vi "SetOrigin.vi"(7 "Available Points in":refnum<vi>, 8 "Error In":errorcluster, 11 "CoordinatteEntry In":T1 {"CaliperSetting"."CaliperEntry"."CaliperType" items=["Distance", "Mid Point", "Perpendicular Projection", "Lines Intersection", "Angle from Horizontal", "Angle from Vertical", "Angle Defined by 3 Points", "Angle Defined by 4 Points", "Bissecting Line", "Mid Line", "Center of Mass", "Area", "Line Fit", "Circle Fit", "Ellipse Fit"]; "OriginPointInfo"."Mode" items=["Horizontal Motion", "Vertical Motion", "Horizontal and Vertical Motion", "Horizontal. Vertical and Angular Motion"]; "AnalysisSetting"."ROI"."Contours"."Type" items=["No Selection", "Point", "Line", "Rectangle", "Oval", "Polygon", "Freehand Region", "Annulus", "Unused2", "Unused3", "Broken Line", "Freehand Line", "Rotated Rectangle"]}) -> (0 "Error Out":errorcluster, 1 "OriginSet?":bool, 3 "CoordinatteEntry Out":T1 {"CaliperSetting"."CaliperEntry"."CaliperType" items=["Distance", "Mid Point", "Perpendicular Projection", "Lines Intersection", "Angle from Horizontal", "Angle from Vertical", "Angle Defined by 3 Points", "Angle Defined by 4 Points", "Bissecting Line", "Mid Line", "Center of Mass", "Area", "Line Fit", "Circle Fit", "Ellipse Fit"]; "OriginPointInfo"."Mode" items=["Horizontal Motion", "Vertical Motion", "Horizontal and Vertical Motion", "Horizontal. Vertical and Angular Motion"]; "AnalysisSetting"."ROI"."Contours"."Type" items=["No Selection", "Point", "Line", "Rectangle", "Oval", "Polygon", "Freehand Region", "Annulus", "Unused2", "Unused3", "Broken Line", "Freehand Line", "Rotated Rectangle"]})   [LabVIEW 2015]
uses:
  Control/CoordinatteEntry.ctl
  Process/Controls/Process_Setting.ctl
  Process/Controls/Process_Type.ctl
  Control/CoordinateAnalysisSetting.ctl
  Control/CoordinateCaliperSetting.ctl
  Caliper/Controls/CaliperDataEntry.ctl
  Caliper/Controls/CaliperType.ctl
  Caliper/Controls/SelectionListEntry.ctl
  Caliper/Controls/SelectionListEntryPointType.ctl
  Caliper/Controls/CaliperResult.ctl
  <vilib>/Utility/miscctls.llb/LVRowAndColumnTypeDef.ctl
panel:
  in  "Mode":u16(ring) items=["Horizontal Motion", "Vertical Motion", "Horizontal and Vertical Motion", "Horizontal. Vertical and Angular Motion"]
  in  "Cancel":bool
  in  "Done":bool
  in  "Available Points":i32(listbox)=5
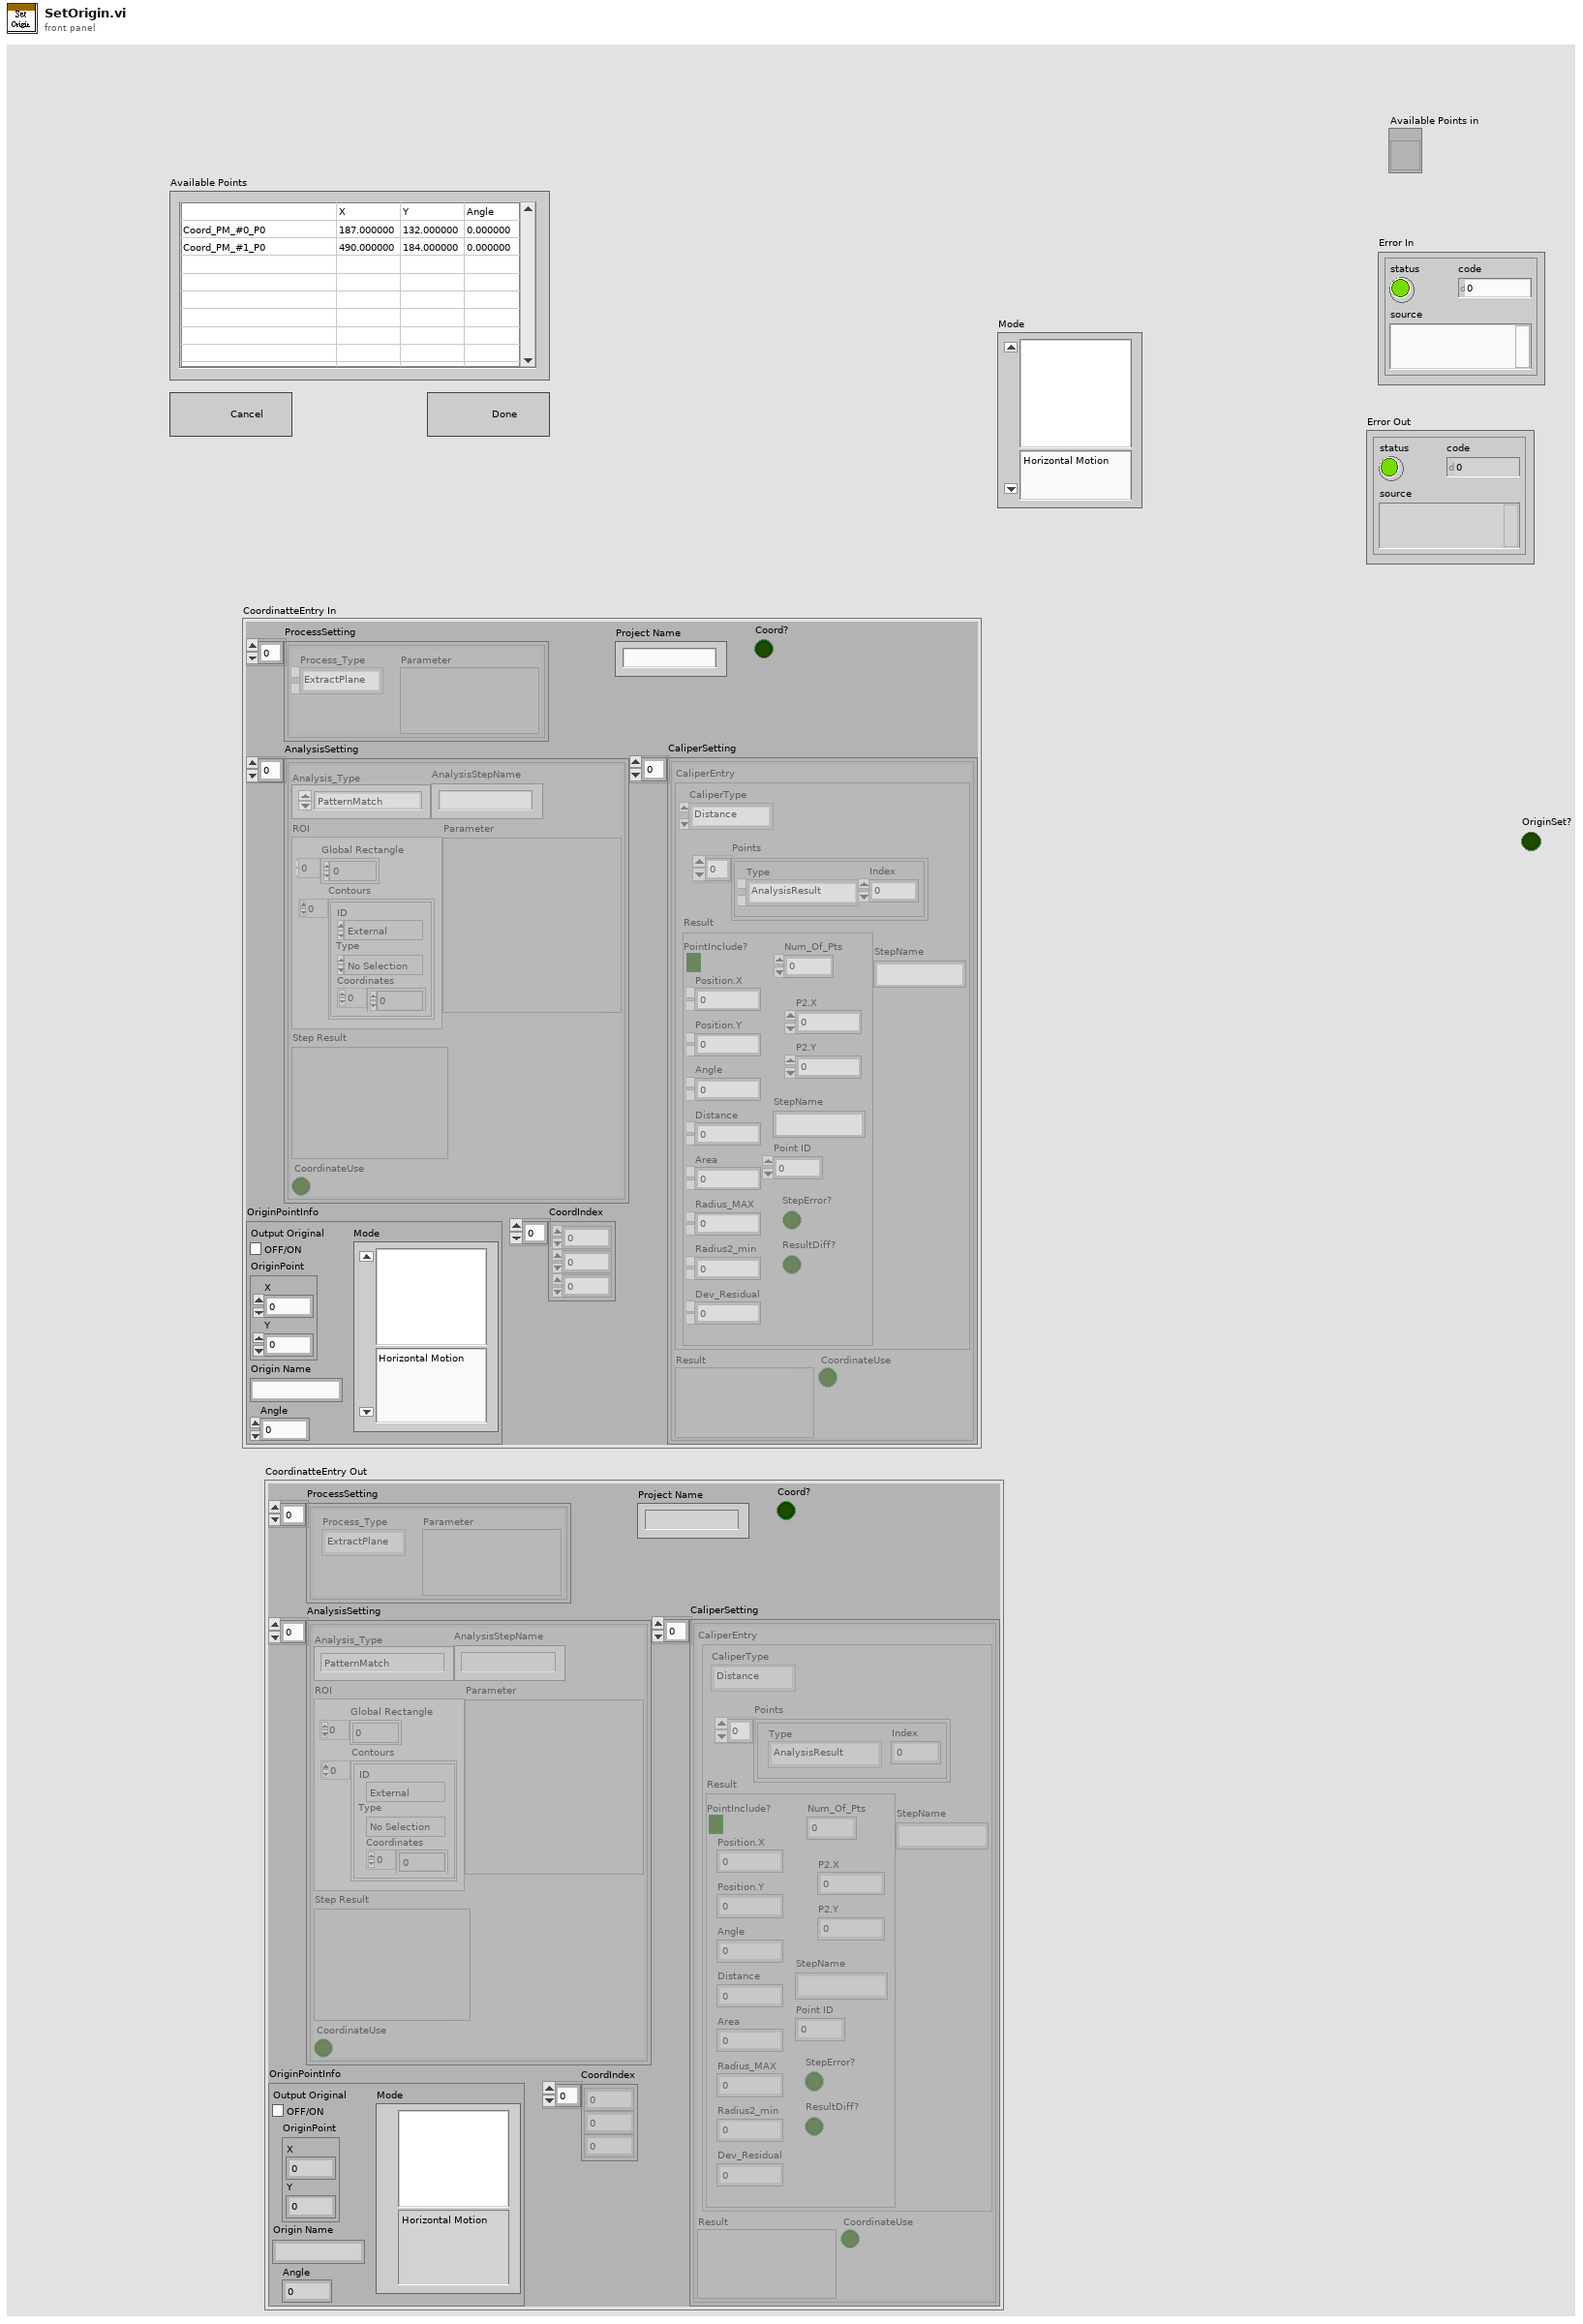
[diagram p1: front panel]
types:
  T1 = typedef "CoordinatteEntry.ctl" = cluster{"ProcessSetting":T2[], "Project Name":string, "AnalysisSetting":T4[], "Coord?":bool, "OriginPointInfo":cluster{"Output Original":bool, "Origin Name":string, "Angle":dbl, "Mode":u16, "OriginPoint":cluster{"X":dbl, "Y":dbl}}, "CaliperSetting":T6[], "CoordIndex":i32[]}
  T2 = typedef "Process_Setting.ctl" = cluster{"Process_Type":T3, "Parameter":variant}
  T3 = typedef "Process_Type.ctl" = enum16{"None", "ExtractPlane", "BinaryMono", "Operators", "GrayMorphology", "Filters", "Lookup Table", "Particle Filter", "Mask"}
  T4 = typedef "CoordinateAnalysisSetting.ctl" = cluster{"Analysis_Type":enum16{"PatternMatch", "Straight Edge"}, "ROI ":T5, "Parameter":variant, "Step Result":variant, "AnalysisStepName":string, "CoordinateUse":bool}
  T5 = typedef "ROI Descriptor" = cluster{"Global Rectangle":i32[], "Contours":cluster{"ID":enum32{"External", "Internal"}, "Type":u32, "Coordinates":i32[]}[]}
  T6 = typedef "CoordinateCaliperSetting.ctl" = cluster{"Result":variant, "CoordinateUse":bool, "CaliperEntry":T7}
  T7 = typedef "CaliperDataEntry.ctl" = cluster{"CaliperType":T8, "Points":T9[], "Result":T11, "StepName":string}
  T8 = typedef "CaliperType.ctl" = u32
  T9 = typedef "SelectionListEntry.ctl" = cluster{"Type":T10, "Index":i32}
  T10 = typedef "SelectionListEntryPointType.ctl" = enum16{"AnalysisResult", "CaliperResult"}
  T11 = typedef "CaliperResult.ctl" = cluster{"PointInclude?":bool, "Num_Of_Pts":u8, "Position.X":dbl, "Position.Y":dbl, "Angle":dbl, "Distance":dbl, "Area":dbl, "Radius_MAX":dbl, "Radius2_min":dbl, "Dev_Residual":dbl, "P2.X":dbl, "P2.Y":dbl, "StepName":string, "Point ID":u8, "StepError?":bool, "ResultDiff?":bool}
  T12 = typedef "LVRowAndColumnTypeDef.ctl" = cluster{"Row":i32, "Column":i32}
  T13 = cluster{"Output Original":bool, "Origin Name":string, "Angle":dbl, "Mode":u16, "OriginPoint":cluster{"X":dbl, "Y":dbl}}
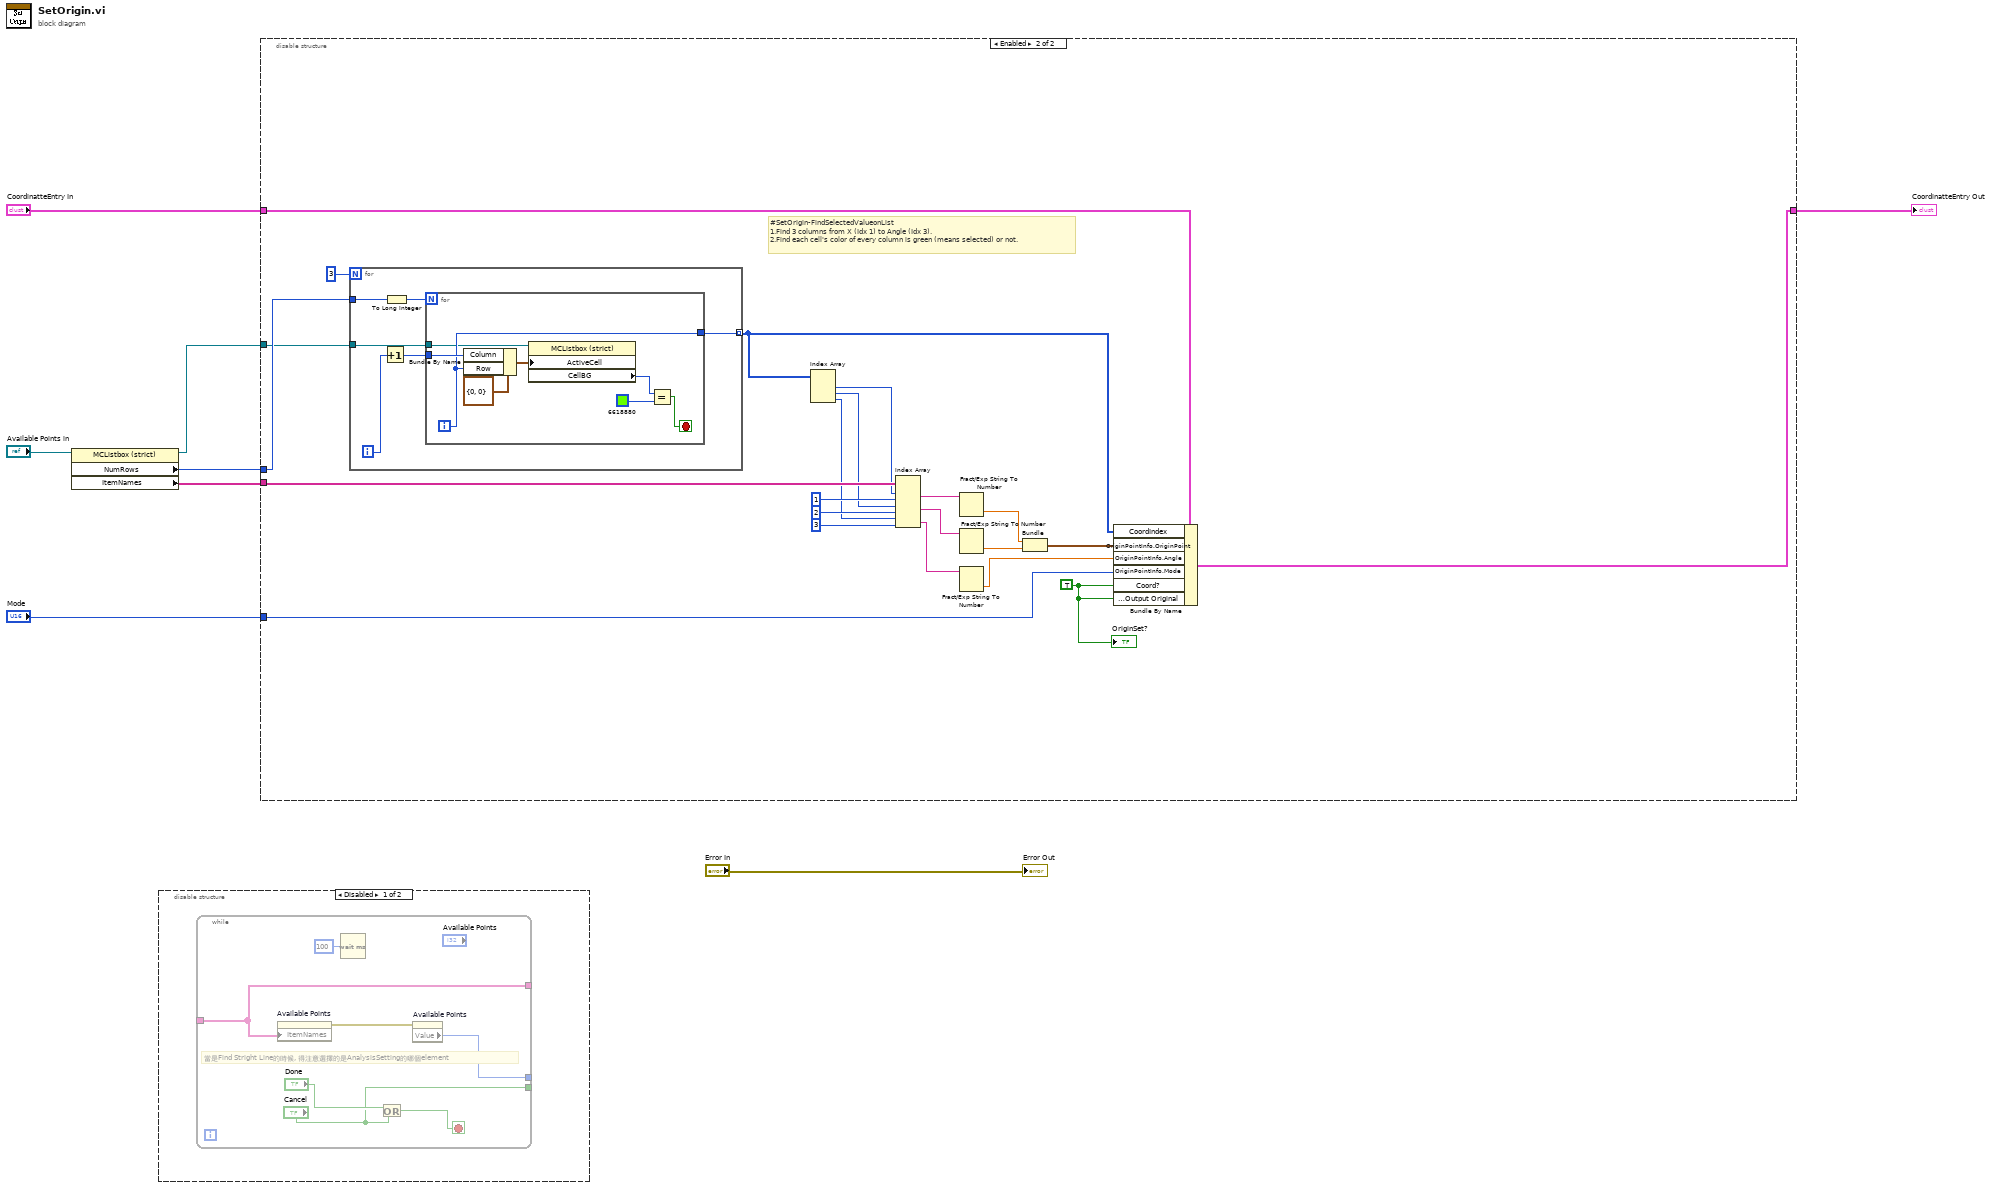
[diagram p0: block diagram]
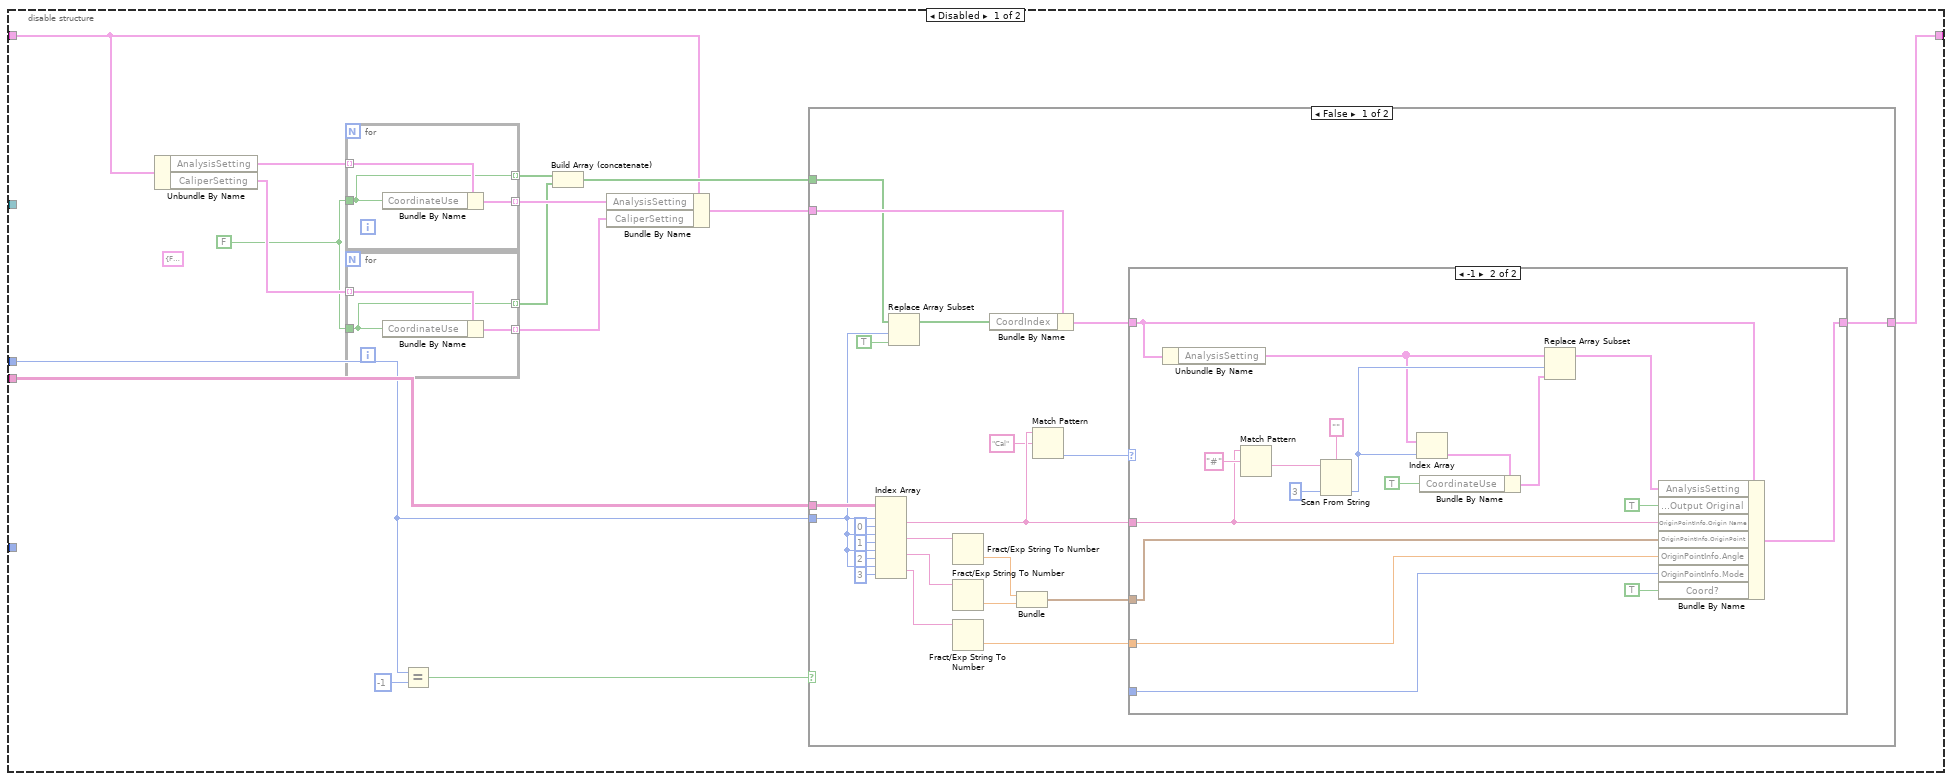
[diagram p2: hidden frame]
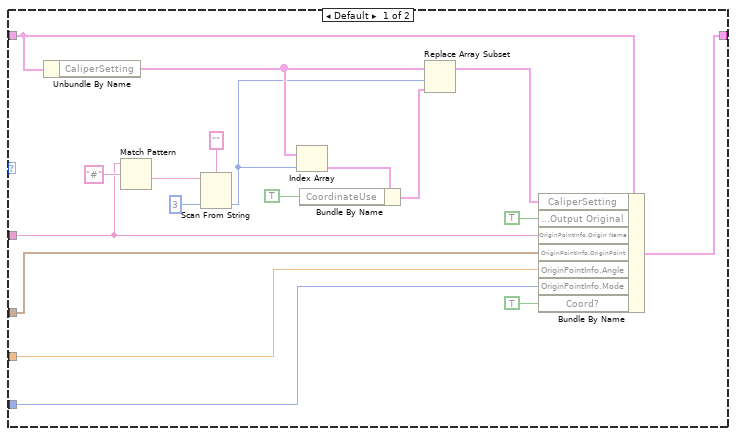
[diagram p3: hidden frame]
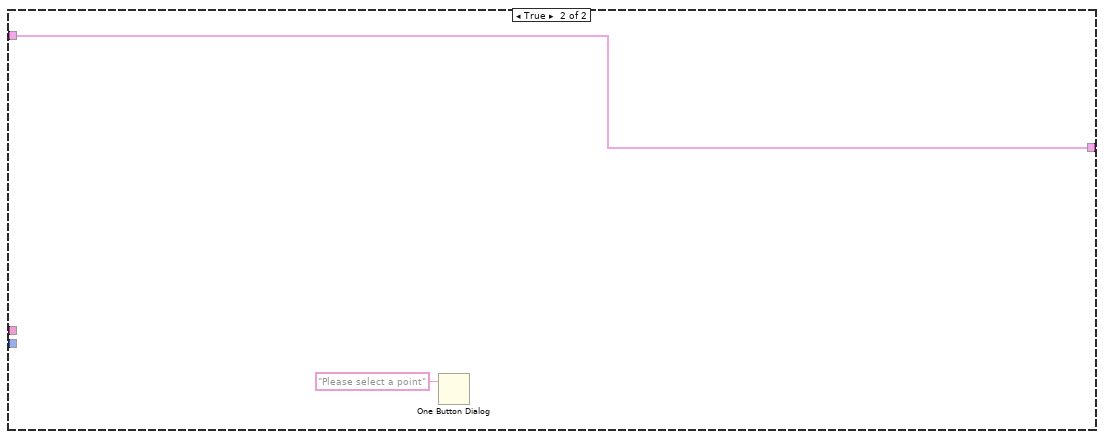
[diagram p4: hidden frame]
diagram:
  n1 = property class="MCListbox (strict)"(reference="Available Points in") -> (reference out=w1:refnum<vi>, "NumRows"=w2:u32, "ItemNames"=w3:string[][])  [unwired: 1 in, 1 out]
  n2 = disable-structure shown="Disabled" {
    frame Disabled {
      n3 = while {
        tunnel: _ -> [w10]
        tunnel: [w14] -> _
        tunnel: [w10] -> _
        tunnel: ["Cancel"] -> _
        stop <- w12 stop-if-true
        # "當是Find Stright Line的時候, 得注意選擇的是AnalysisSetting的哪個element"
        n4 = property on="Available Points" class="MCListbox (strict)"("ItemNames"=w10) -> (error out=w15:errorcluster)  [unwired: 2 in, 1 out]
        n5 = Wait (ms)(milliseconds to wait=u32 100) -> ()  [unwired: 1 out]
        n6 = Or(x="Done", y="Cancel") -> (x .or. y?=w12:bool)
        n7 = property on="Available Points" class="MCListbox (strict)"(error in=w15) -> ("Value"=w14:i32)  [unwired: 1 in, 2 out]
      }
    }
    frame Enabled {
    }
  }
  n8 = disable-structure shown="Enabled" {
    disable-tunnel: w3 -> [w30 w119]
    disable-tunnel: [w29 w108] -> w6
    disable-tunnel: w2 -> [w24 w101]
    disable-tunnel: "CoordinatteEntry In" -> [w16 w106]
    disable-tunnel: "Mode" -> [_ w107]
    disable-tunnel: w1 -> [_ w98]
    frame Disabled {
      w21 = FALSE
      (unwired) T13 {"Output Original"=FALSE, "Origin Name"="", "Angle"=0.0, "Mode"=0, "OriginPoint"={"X"=0.0, "Y"=0.0}} ("OriginPointInfo")
      n9 = Unbundle By Name(w16) -> ("AnalysisSetting"=w27:T4[], "CaliperSetting"=w22:T6[])
      n10 = for {
        tunnel: w27 -> [w36] mode=indexing
        tunnel: [w35] -> w25 mode=indexing
        tunnel: w21 -> [w34]
        tunnel: [w34] -> w19 mode=indexing
        n11 = Bundle By Name(cluster=w36, "CoordinateUse"=w34) -> (w35:T4)
      }
      n12 = for {
        tunnel: w22 -> [w33] mode=indexing
        tunnel: [w32] -> w20 mode=indexing
        tunnel: w21 -> [w31]
        tunnel: [w31] -> w18 mode=indexing
        n13 = Bundle By Name(cluster=w33, "CoordinateUse"=w31) -> (w32:T6)
      }
      n14 = Equal?(x=w24, y=-1) -> (x = y?=w28:bool)
      n15 = Build Array (concatenate)(w19, w18) -> (w17:bool[])
      n16 = Bundle By Name(cluster=w16, "AnalysisSetting"=w25, "CaliperSetting"=w20) -> (w26:T1)
      n17 = case shown="False" w28 {
        tunnel: w26 -> [w40 w97]
        tunnel: w30 -> [w59 _]
        tunnel: w24 -> [w43 _]
        tunnel: [w41 w97] -> w29
        tunnel: w17 -> [w37 _]
        frame False {
          n18 = Index Array(array=w59, index (row) #1=w43, index (col) #1=0 ("disabled index (col)"), index (row) #2=w43, index (col) #2=1 ("disabled index (col)"), index (row) #3=w43, index (col) #3=2 ("disabled index (col)"), index (row) #4=w43, index (col) #4=3 ("disabled index (col)")) -> (element #1=w46:string, element #2=w54:string, element #3=w53:string, element #4=w52:string)
          n19 = Replace Array Subset(array=w37, new element=TRUE ("new element/subarray"), index=w43) -> (w38:bool[])
          n20 = Fract/Exp String To Number(string=w54) -> (number=w50:dbl)  [unwired: 3 in, 1 out]
          n21 = Fract/Exp String To Number(string=w53) -> (number=w49:dbl)  [unwired: 3 in, 1 out]
          n22 = Fract/Exp String To Number(string=w52) -> (number=w51:dbl)  [unwired: 3 in, 1 out]
          n23 = Bundle By Name(cluster=w40, "CoordIndex"=w38) -> (w39:T1)
          n24 = Bundle(w50, w49) -> (w47:cluster{dbl, dbl})  [unwired: 1 in]
          n25 = Match Pattern(string=w46, regular expression="Cal") -> (offset past match=w44:i32)  [unwired: 1 in, 3 out]
          n26 = case shown="-1" w44 {
            tunnel: w51 -> [w74 w79]
            tunnel: [w77 w91] -> w41
            tunnel: [w76 w83] -> w48
            tunnel: w47 -> [w75 w80]
            tunnel: w46 -> [w66 w81]
            tunnel: w39 -> [w73 w84]
            frame Default {
              n27 = Unbundle By Name(w73) -> ("CaliperSetting"=w64:T6[])
              n28 = Match Pattern(string=w66, regular expression="#") -> (after substring=w69:string)  [unwired: 1 in, 3 out]
              n29 = Scan From String(format string="", input string=w69, default 1=3 ("disabled index (col)")) -> (output 1=w61:i32)  [unwired: 2 in, 3 out]
              n30 = Index Array(array=w64, index=w61) -> (element=w63:T6)
              n31 = Bundle By Name(cluster=w63, "CoordinateUse"=TRUE ("Original Point.Output Original")) -> (w62:T6)
              n32 = Replace Array Subset(array=w64, new element=w62, index=w61) -> (w72:T6[])
              n33 = Bundle By Name(cluster=w73, "CaliperSetting"=w72, "OriginPointInfo.Output Original"=TRUE, "OriginPointInfo.Origin Name"=w66, "OriginPointInfo.OriginPoint"=w75, "OriginPointInfo.Angle"=w74, "OriginPointInfo.Mode"=w76, "Coord?"=TRUE) -> (w77:T1)
            }
            frame -1 {
              n34 = Unbundle By Name(w84) -> ("AnalysisSetting"=w85:T4[])
              n35 = Match Pattern(string=w81, regular expression="#") -> (after substring=w89:string)  [unwired: 1 in, 3 out]
              n36 = Scan From String(format string="", input string=w89, default 1=3 ("disabled index (col)")) -> (output 1=w86:i32)  [unwired: 2 in, 3 out]
              n37 = Index Array(array=w85, index=w86) -> (element=w95:T4)
              n38 = Bundle By Name(cluster=w95, "CoordinateUse"=TRUE ("Original Point.Output Original")) -> (w93:T4)
              n39 = Replace Array Subset(array=w85, new element=w93, index=w86) -> (w92:T4[])
              n40 = Bundle By Name(cluster=w84, "AnalysisSetting"=w92, "OriginPointInfo.Output Original"=TRUE, "OriginPointInfo.Origin Name"=w81, "OriginPointInfo.OriginPoint"=w80, "OriginPointInfo.Angle"=w79, "OriginPointInfo.Mode"=w83, "Coord?"=TRUE) -> (w91:T1)
            }
          }
        }
        frame True {
          n41 = One Button Dialog(message="Please select a point") -> ()  [unwired: 1 in, 1 out]
        }
      }
    }
    frame Enabled {
      w99 = TRUE ("Coord?")
      # "#SetOrigin-FindSelectedValueonList\n1.Find 3 columns from X (Idx 1) to Angle (Idx 3).\n2.Find each cell's color of every column is green (means selected) or not."
      n42 = for {
        N: 3 -> [_]
        tunnel: w101 -> [w125]
        tunnel: [w121] -> w100 mode=indexing
        tunnel: w98 -> [w120]
        i -> [w124]
        n43 = Increment(x=w124) -> (x+1=w122:i32)
        n44 = To Long Integer(number=w125) -> (32bit integer=w123:i32)
        n45 = for {
          N: w123 -> [_]
          tunnel: w122 -> [w132]
          tunnel: [w128] -> w121
          tunnel: w120 -> [w126]
          i -> [w128]
          stop <- w127 stop-if-true
          n46 = Bundle By Name(cluster=T12 {"Row"=0, "Column"=0} ("Active Cell:Active Cell"), "Column"=w132, "Row"=w128) -> (w131:T12)
          n47 = property class="MCListbox (strict)"(reference=w126, "ActiveCell"=w131) -> ("CellBG"=w130:u32)  [unwired: 1 in, 2 out]
          n48 = Equal?(x=w130, y=u32 6618880) -> (x = y?=w127:bool)
        }
      }
      n49 = Index Array(array=w100) -> (element #1=w105:i32, element #2=w104:i32, element #3=w103:i32)  [unwired: 3 in]
      n50 = Index Array(array=w119, index (row) #1=w105, index (col) #1=1 ("disabled index (col)"), index (row) #2=w104, index (col) #2=2 ("disabled index (col)"), index (row) #3=w103, index (col) #3=3 ("index (col)")) -> (element #1=w113:string, element #2=w112:string, element #3=w111:string)
      n51 = Fract/Exp String To Number(string=w113) -> (number=w115:dbl)  [unwired: 3 in, 1 out]
      n52 = Fract/Exp String To Number(string=w112) -> (number=w114:dbl)  [unwired: 3 in, 1 out]
      n53 = Fract/Exp String To Number(string=w111) -> (number=w109:dbl)  [unwired: 3 in, 1 out]
      n54 = Bundle(w115, w114) -> (w110:cluster{dbl, dbl})  [unwired: 1 in]
      n55 = Bundle By Name(cluster=w106, "CoordIndex"=w100, "OriginPointInfo.OriginPoint"=w110, "OriginPointInfo.Angle"=w109, "OriginPointInfo.Mode"=w107, "Coord?"=w99, "OriginPointInfo.Output Original"=w99) -> (w108:T1)
      "OriginSet?" <- w99
    }
  }
  "CoordinatteEntry Out" <- w6
  "Error Out" <- "Error In"
